vi "改变位图.vi"(2 "Exit Event":refnum<user-event>) -> ()   [LabVIEW 2018]
doc: "This example shows how to create an image in IMAQ Vision, read an image file from disk, and display it in an image window."
uses:
  <vilib>/userdefined/High Color/IMAQdx.ctl
  <vilib>/vision/Image Controls.llb/IMAQ Image.ctl
  <vilib>/vision/driver/IMAQdx.llb/IMAQdx Acquisition Mode.ctl
  <vilib>/vision/NI_Vision_Development_Module.lvlib
  <vilib>/vision/driver/NI_Vision_Acquisition_Software.lvlib
panel:
  in  "stop":bool
  in  "开始":bool
  in  "静态/实时":bool
  in  "IMAQdx Session":T1
  in  "Bit-depth":i8=8 min=1 max=8 step=1
  in  "Save Button":bool
  out "原图":T2(plugin-control)
  out "处理后图像":T2(plugin-control)
  # "Select the image-depth below and observe changes in the image.\nHit 'stop' to exit program."
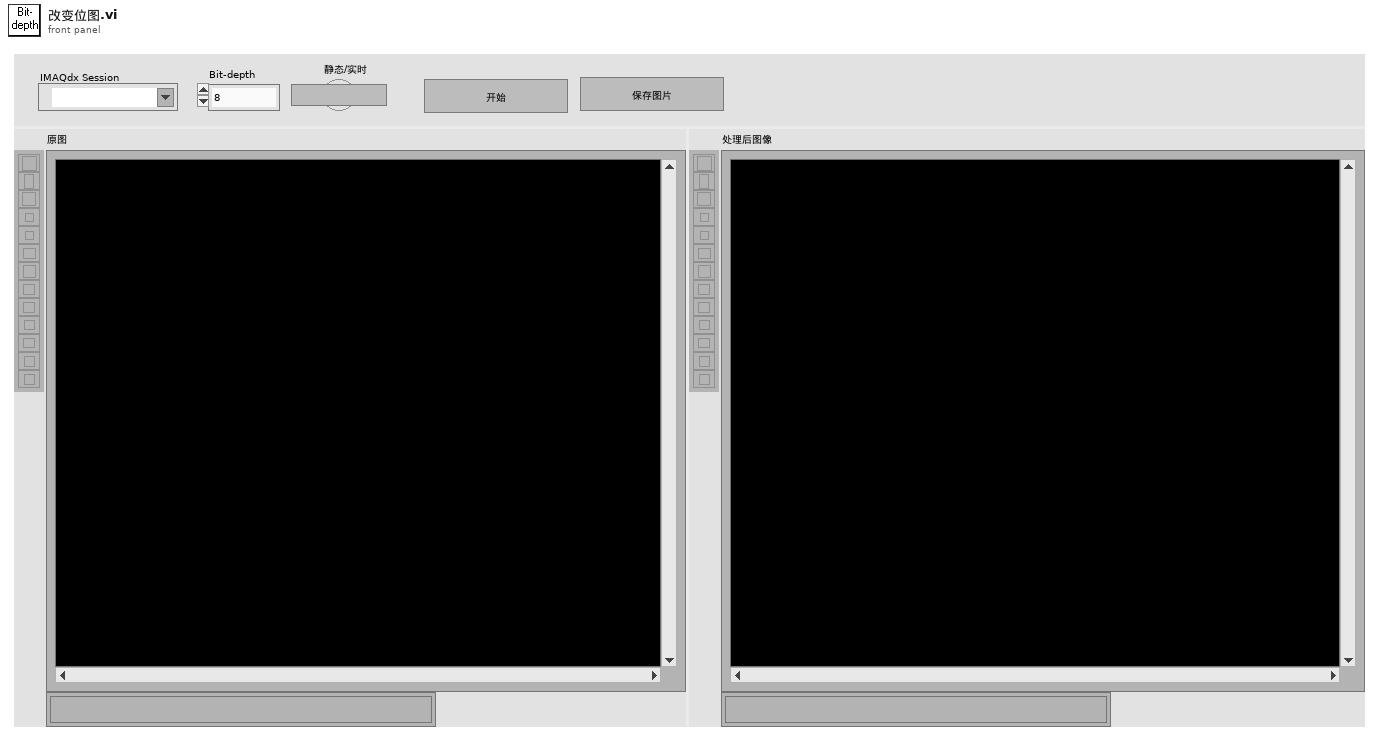
[diagram p1: front panel]
types:
  T1 = typedef "IMAQdx.ctl" = refnum<k21>
  T2 = typedef "IMAQ Image.ctl" = refnum<image>
  T3 = enum8{"Enabled", "Disabled", "Disabled and Grayed Out"}
  T4 = typedef "NI_Vision_Acquisition_Software.lvlib/IMAQdx Acquisition Mode.ctl" = enum32{"One Shot", "Continuous"}
  T5 = typedef "Image Type" = u32
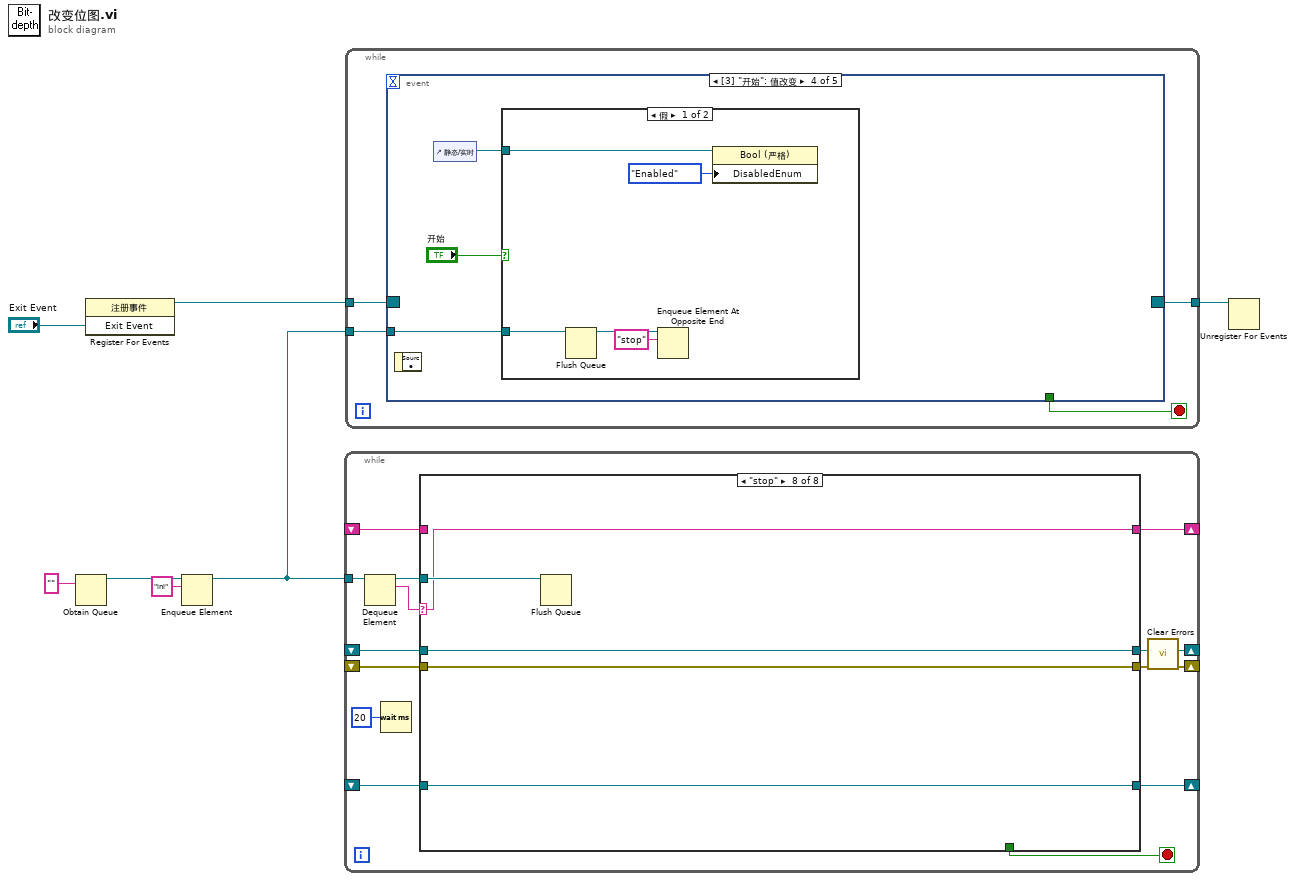
[diagram p0: block diagram]
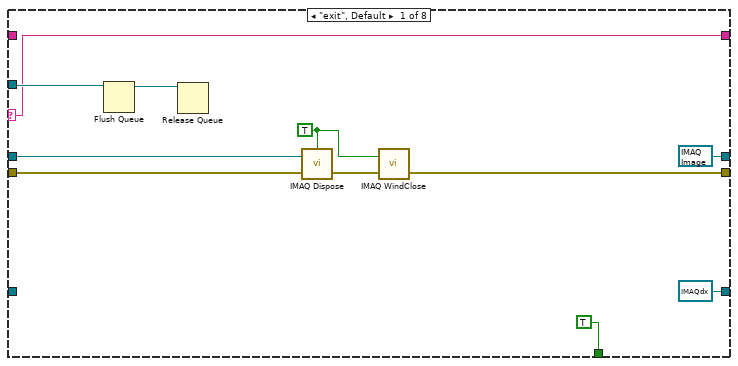
[diagram p2: hidden frame]
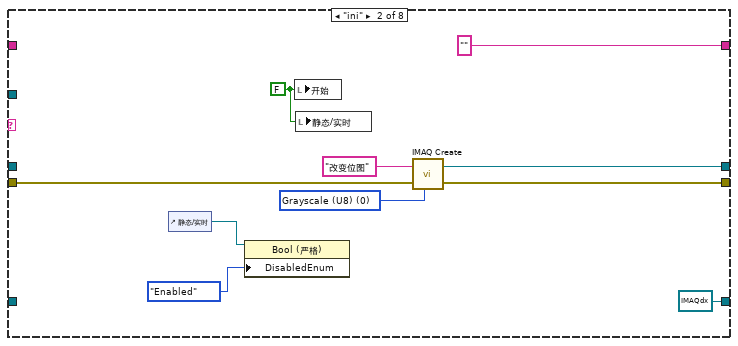
[diagram p3: hidden frame]
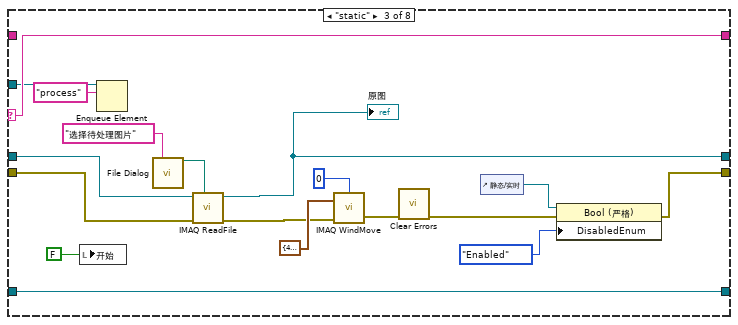
[diagram p4: hidden frame]
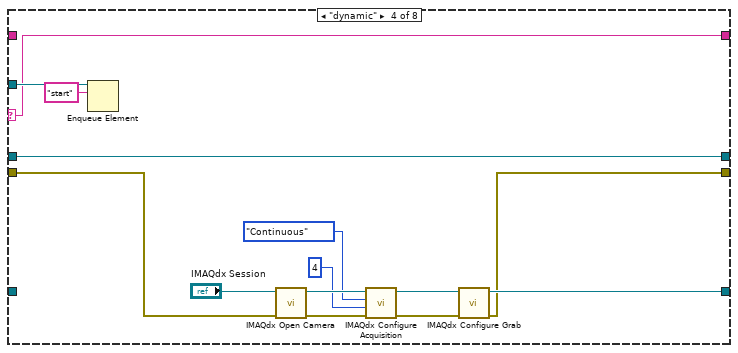
[diagram p5: hidden frame]
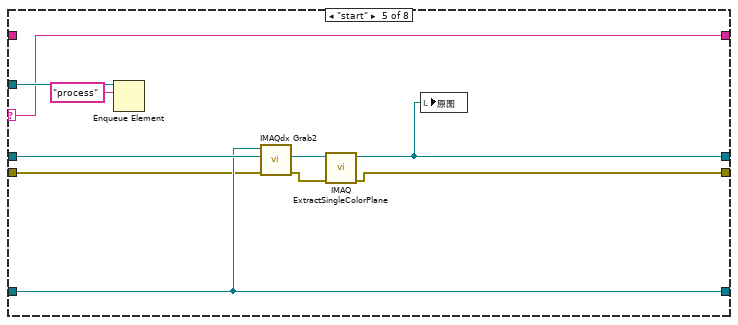
[diagram p6: hidden frame]
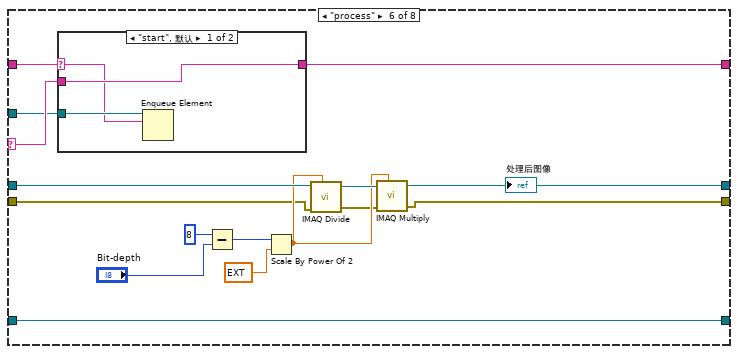
[diagram p7: hidden frame]
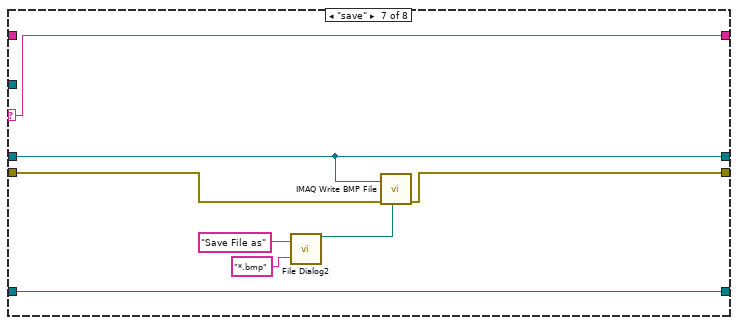
[diagram p9: hidden frame]
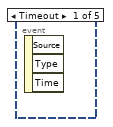
[diagram p10: hidden frame]
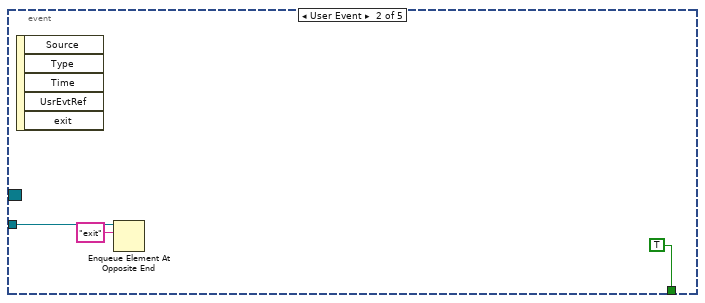
[diagram p11: hidden frame]
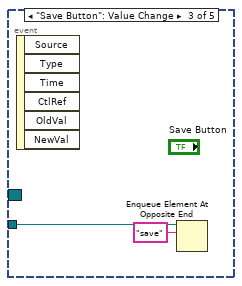
[diagram p12: hidden frame]
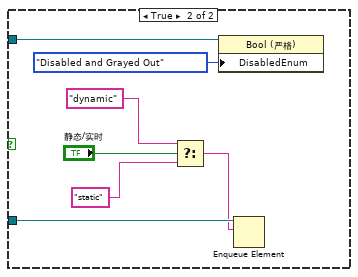
[diagram p13: hidden frame]
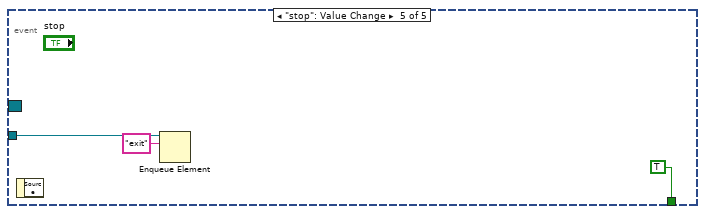
[diagram p14: hidden frame]
diagram:
  n1 = Obtain Queue(element data type="") -> (queue out=w3:refnum<queue>)  [unwired: 4 in, 2 out]
  n2 = register-events("Exit Event") -> (reference out=w6:refnum<event-registration>)  [unwired: 2 in, 1 out]
  n3 = Enqueue Element(queue=w3, element="ini") -> (queue out=w1:refnum<queue>)  [unwired: 2 in, 2 out]
  n4 = while {
    tunnel: w1 -> [w21]
    shift-right: [w17] -> _
    shift-left: _ -> [w16]
    shift-right: [w15] -> _
    shift-left: _ -> [w14]
    shift-right: [w13] -> _
    shift-left: _ -> [w12]
    shift-right: [w9] -> _
    shift-left: _ -> [w11]
    stop <- w18 stop-if-true
    n5 = Dequeue Element(queue=w21) -> (queue out=w19:refnum<queue>, element=w20:string)  [unwired: 2 in, 2 out]
    n6 = Wait (ms)(milliseconds to wait=u32 20 ("等待时间（毫秒）")) -> ()  [unwired: 1 out]
    n7 = case shown="\"stop\"" w20 {
      selector: w20 -> [w24 _ w55 w71 w79 w90 w107 w114]
      tunnel: w19 -> [w32 _ w54 w73 w80 w88 _ w117]
      tunnel: [TRUE _ _ _ _ _ _ _] -> w18
      tunnel: [T2 refnum ("New Image") w38 w43 w74 w82 w100 w109 w116] -> w17
      tunnel: w16 -> [w27 _ w51 w74 w83 w99 w109 w116]
      tunnel: [T1 refnum ("Session Out") T1 refnum ("Session Out") w56 w63 w81 w92 w108 w115] -> w15
      tunnel: w14 -> [_ _ w56 _ w81 w92 w108 w115]
      tunnel: [w24 "" w55 w71 w79 w89 w107 w114] -> w13
      tunnel: w12 -> [_ _ _ _ _ w91 _ _]
      tunnel: w11 -> [w23 w34 w46 w61 w77 w87 w106 w113]
      tunnel: [w22 w33 w45 w62 w75 w85 w105 w113] -> w10
      frame "exit", Default {
        w28 = TRUE ("All Images? (No)")
        n8 = Flush Queue(queue=w32) -> (queue out=w31:refnum<queue>)  [unwired: 1 in, 2 out]
        n9 = Release Queue(queue=w31) -> ()  [unwired: 2 in, 3 out]
        n10 = call "IMAQ Dispose"("All Images? (No)"=w28, "Image"=w27, "error in (no error)"=w23) -> ("error out"=w29:errorcluster)  [unwired: 3 in]
        n11 = call "IMAQ WindClose"("Close All Windows (False)"=w28, "error in (no error)"=w29) -> ("error out"=w22:errorcluster)  [unwired: 4 in]
      }
      frame "ini" {
        w35 = FALSE ("开始")
        w39 = T5 0 items=["Grayscale (U8)", "Grayscale (I16)", "Grayscale (SGL)", "Complex (CSG)", "RGB (U32)", "HSL (U32)", "RGB (U64)", "Grayscale (U16)"] ("Image Type")
        n12 = control-ref of="静态/实时"() -> (w37:refnum<vi>)
        n13 = property class="Bool (严格)"(reference=w37, "DisabledEnum"=T3."Enabled" ("Disabled")) -> ()  [unwired: 1 in, 2 out]
        n14 = local write "开始"(w35) -> ()
        n15 = local write "静态/实时"(w35) -> ()
        n16 = call "IMAQ Create"("Image Name"="改变位图", "Image Type"=w39, "error in (no error)"=w34) -> ("New Image"=w38:T2, "error out"=w33:errorcluster)  [unwired: 2 in]
      }
      frame "static" {
        n17 = local write "开始"(FALSE ("开始")) -> ()
        n18 = Enqueue Element(queue=w54, element="process") -> ()  [unwired: 2 in, 3 out]
        n19 = call "File Dialog"("prompt"="选择待处理图片") -> ("selected path"=w60:path)  [unwired: 11 in, 3 out]
        n20 = call "IMAQ ReadFile"("File Path"=w60, "error in (no error)"=w46, "Image"=w51) -> ("error out"=w44:errorcluster, "Image Out"=w43:T2)  [unwired: 4 in, 3 out]
        "原图" <- w43
        n21 = call "IMAQ WindMove"("Window Number (0...15)"=0, "Coordinates (screen)"=cluster{"X Position":i32, "Y Position":i32} {"X Position"=40, "Y Position"=400}, "error in (no error)"=w44) -> ("error out"=w48:errorcluster)  [unwired: 2 in, 1 out]
        n22 = call <vilib>:"Clear Errors.vi"("error in (no error)"=w48) -> ("error out"=w47:errorcluster)  [unwired: 5 in, 1 out]
        n23 = control-ref of="静态/实时"() -> (w50:refnum<vi>)
        n24 = property class="Bool (严格)"(reference=w50, error in=w47, "DisabledEnum"=T3."Enabled" ("Disabled")) -> (error out=w45:errorcluster)  [unwired: 1 out]
      }
      frame "dynamic" {
        n25 = Enqueue Element(queue=w73, element="start") -> ()  [unwired: 2 in, 3 out]
        n26 = call <vilib>:"IMAQdx Open Camera.vi"("error in"=w61, "Session In"="IMAQdx Session") -> ("error out"=w65:errorcluster, "Session Out"=w70:T1)  [unwired: 8 in]
        n27 = call <vilib>:"IMAQdx Configure Acquisition.vi"("error in"=w65, "Number of Buffers"=u32 4, "Continuous?"=IMAQdx_Acquisition_Mode."Continuous", "Session In"=w70) -> ("error out"=w66:errorcluster, "Session Out"=w67:T1)  [unwired: 6 in]
        n28 = call <vilib>:"IMAQdx Configure Grab.vi"("error in"=w66, "Session In"=w67) -> ("error out"=w62:errorcluster, "Session Out"=w63:T1)  [unwired: 8 in]
      }
      frame "start" {
        n29 = Enqueue Element(queue=w80, element="process") -> ()  [unwired: 2 in, 3 out]
        n30 = call <vilib>:"IMAQdx Grab2.vi"("error in"=w77, "Image In"=w83, "Session In"=w81) -> ("error out"=w76:errorcluster, "Image Out"=w84:T2)  [unwired: 5 in, 2 out]
        n31 = call "IMAQ ExtractSingleColorPlane"("error in (no error)"=w76, "Image Src"=w84) -> ("error out"=w75:errorcluster, "Image Dst Out"=w82:T2)  [unwired: 8 in]
        n32 = local write "原图"(w82) -> ()
      }
      frame "process" {
        n33 = case shown="\"start\", 默认" w91 {
          selector: w91 -> [w101 _]
          tunnel: w90 -> [w102 w104]
          tunnel: [w102 w104] -> w89
          tunnel: w88 -> [w103 _]
          frame "start", Default {
            n34 = Enqueue Element(queue=w103, element=w101) -> ()  [unwired: 2 in, 3 out]
          }
          frame "static" {
          }
        }
        n35 = Subtract(x=i8 8, y="Bit-depth") -> (x-y=w96:i8)
        n36 = Scale By Power Of 2(n=w96, x=ext 1.0) -> (x*2^n=w93:ext)
        n37 = call "IMAQ Divide"("Image Src A"=w99, "Constant"=w93, "error in (no error)"=w87) -> ("Image Dst Out"=w94:T2, "error out"=w86:errorcluster)  [unwired: 4 in]
        n38 = call "IMAQ Multiply"("Image Src A"=w94, "Constant"=w93, "error in (no error)"=w86) -> ("Image Dst Out"=w100:T2, "error out"=w85:errorcluster)  [unwired: 4 in]
        "处理后图像" <- w100
      }
      frame "save" {
        n39 = call "File Dialog2"("prompt"="Save File as", "pattern (all files)"="*.bmp" ("pattern")) -> ("selected path"=w112:path)  [unwired: 10 in, 3 out]
        n40 = call "IMAQ Write BMP File"("error in (no error)"=w106, "File Path"=w112, "Image"=w109) -> ("error out"=w105:errorcluster)  [unwired: 5 in]
      }
      frame "stop" {
        n41 = Flush Queue(queue=w117) -> ()  [unwired: 1 in, 3 out]
      }
    }
    n42 = call <vilib>:"Clear Errors.vi"("error in (no error)"=w10) -> ("error out"=w9:errorcluster)  [unwired: 5 in, 1 out]
  }
  n43 = while {
    tunnel: w6 -> [w121]
    tunnel: [w120] -> w5
    tunnel: w1 -> [w118]
    stop <- w119 stop-if-true
    n44 = event shown="[3] \"开始\": 值改变" {
      selector: w121 -> [_ _ _ _ _]
      dyn-events: [_ _ _ _ _] -> w120
      timeout: _ -> [_ _ _ _ _]
      tunnel: [_ TRUE _ _ TRUE] -> w119
      tunnel: w118 -> [_ w123 w126 w129 w143]
      event Timeout {
        n45 = event-data() -> ()  [unwired: 1 in, 3 out]
      }
      event User Event {
        n46 = event-data() -> ()  [unwired: 1 in, 5 out]
        n47 = Enqueue Element At Opposite End(queue=w123, element="exit") -> ()  [unwired: 2 in, 3 out]
      }
      event "Save Button": Value Change {
        n48 = event-data() -> ()  [unwired: 1 in, 6 out]
        n49 = Enqueue Element At Opposite End(queue=w126, element="save") -> ()  [unwired: 2 in, 3 out]
      }
      event "开始": Value Change {
        n50 = event-data() -> ()  [unwired: 1 in, 1 out]
        n51 = control-ref of="静态/实时"() -> (w127:refnum<vi>)
        n52 = case shown="假" "开始" {
          tunnel: w129 -> [w134 w141]
          tunnel: w127 -> [w130 w136]
          frame False {
            n53 = Flush Queue(queue=w134) -> (queue out=w133:refnum<queue>)  [unwired: 1 in, 2 out]
            n54 = Enqueue Element At Opposite End(queue=w133, element="stop") -> ()  [unwired: 2 in, 3 out]
            n55 = property class="Bool (严格)"(reference=w130, "DisabledEnum"=T3."Enabled" ("Disabled")) -> ()  [unwired: 1 in, 2 out]
          }
          frame True {
            n56 = Select(t="dynamic" ("f"), s="静态/实时", f="static" ("element")) -> (s? t:f=w139:string)
            n57 = property class="Bool (严格)"(reference=w136, "DisabledEnum"=T3."Disabled and Grayed Out" ("Disabled")) -> ()  [unwired: 1 in, 2 out]
            n58 = Enqueue Element(queue=w141, element=w139) -> ()  [unwired: 2 in, 3 out]
          }
        }
      }
      event "stop": Value Change {
        n59 = event-data() -> ()  [unwired: 1 in, 1 out]
        n60 = Enqueue Element(queue=w143, element="exit") -> ()  [unwired: 2 in, 3 out]
      }
    }
  }
  n61 = Unregister For Events(event registration refnum=w5) -> ()  [unwired: 1 in, 1 out]
